vi "PositionToReceivePassSkill.vi"(5 "first call":bool, 7 "Striker/2ndStriker":enum16{"2ndStriker", "Striker"}(ring), 8 "error in (no error)":errorcluster, 9 "Robot":refnum<class "Robot.lvclass">, 10 "Game":refnum<class "Game.lvclass">, 11 "PositionToReceivePassSkill in":refnum<class "PositionToReceivePassSkill.lvclass">) -> (0 "error out":errorcluster, 2 "Robot out":refnum<class "Robot.lvclass">, 3 "PositionToReceivePassSkill out":refnum<class "PositionToReceivePassSkill.lvclass">)   [LabVIEW 2018, in "PositionToReceivePassSkill.lvclass"]
uses:
  PositionToReceivePassSkill.lvclass
  Game_class/Game.lvclass
  Robot_class/Robot.lvclass
  Game_class/Game.lvclass/Game.ctl
  Parameters_class/Parameters.lvclass/Parameters.ctl
  Team_class/Team.lvclass/Team.ctl
  Object_class/Object.lvclass/Object.ctl
  Robot_class/Robot.lvclass/Robot.ctl
  Robot_class/roles.ctl
  Utilities_class/Utilities.lvclass
  Object_class/Read x.vi
  Object_class/Read y.vi
  Robot_class/Read role.vi
  Robot_class/Read orientation.vi
  Game_class/Read OffensiveTeam.vi
  Game_class/Read FieldRef.vi
  Team_class/Read RobotRef.vi
  Game_class/Read Parameters.lvclass.vi
  Parameters_class/Read AttakingOurselves.vi
  Robot_class/Write dest_x.vi
  Robot_class/Write dest_y.vi
  Robot_class/Write dest_orientation.vi
  Ally_class/Ally.lvclass
  Field_class/Field.lvclass
  Parameters_class/Parameters.lvclass
panel:
  in  "Field defense":dbl[](array[numeric])
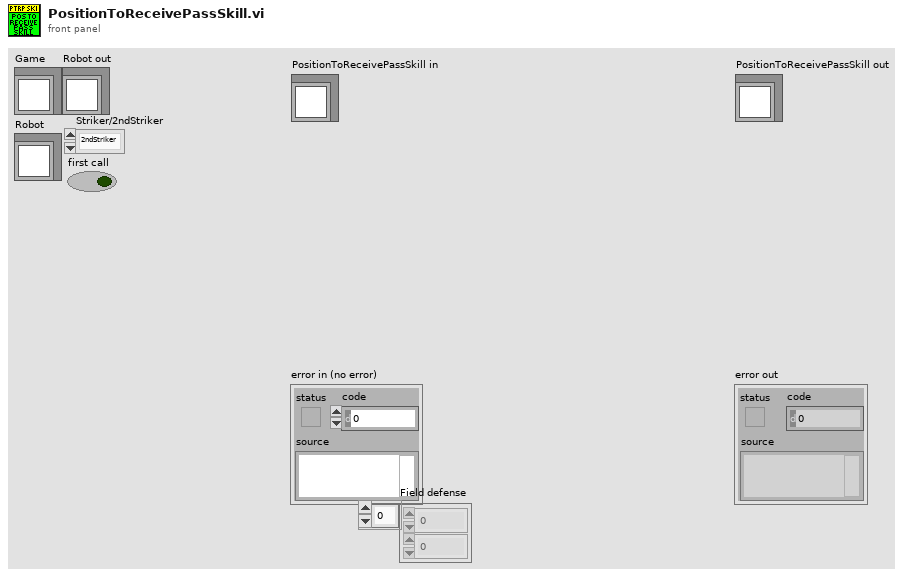
[diagram p1: front panel]
types:
  T1 = typedef "roles.ctl" = enum16{"PrepareRollToPassRoller", "PrepareRollToPassReceiver", "SimplePassRoll", "SimplePassRollReceiver", "PenaltyDefense", "PreparePassReceiver 2", "PreparePassReceiver 1", "PassObserver", "Timeout", "Goto", "ZigZag", "None", "BallOutOfField", "DefenderArea", "Duelist", "AttackerStop", "FollowAttacker", "KeeperRole", "KickPenalty", "AttackerAimGoal", "AttackerBlock", "Marker", "Halt", "Shoot", "PassKicker", "PassReceiver", "TestRole", "PenaltyAttacker"}
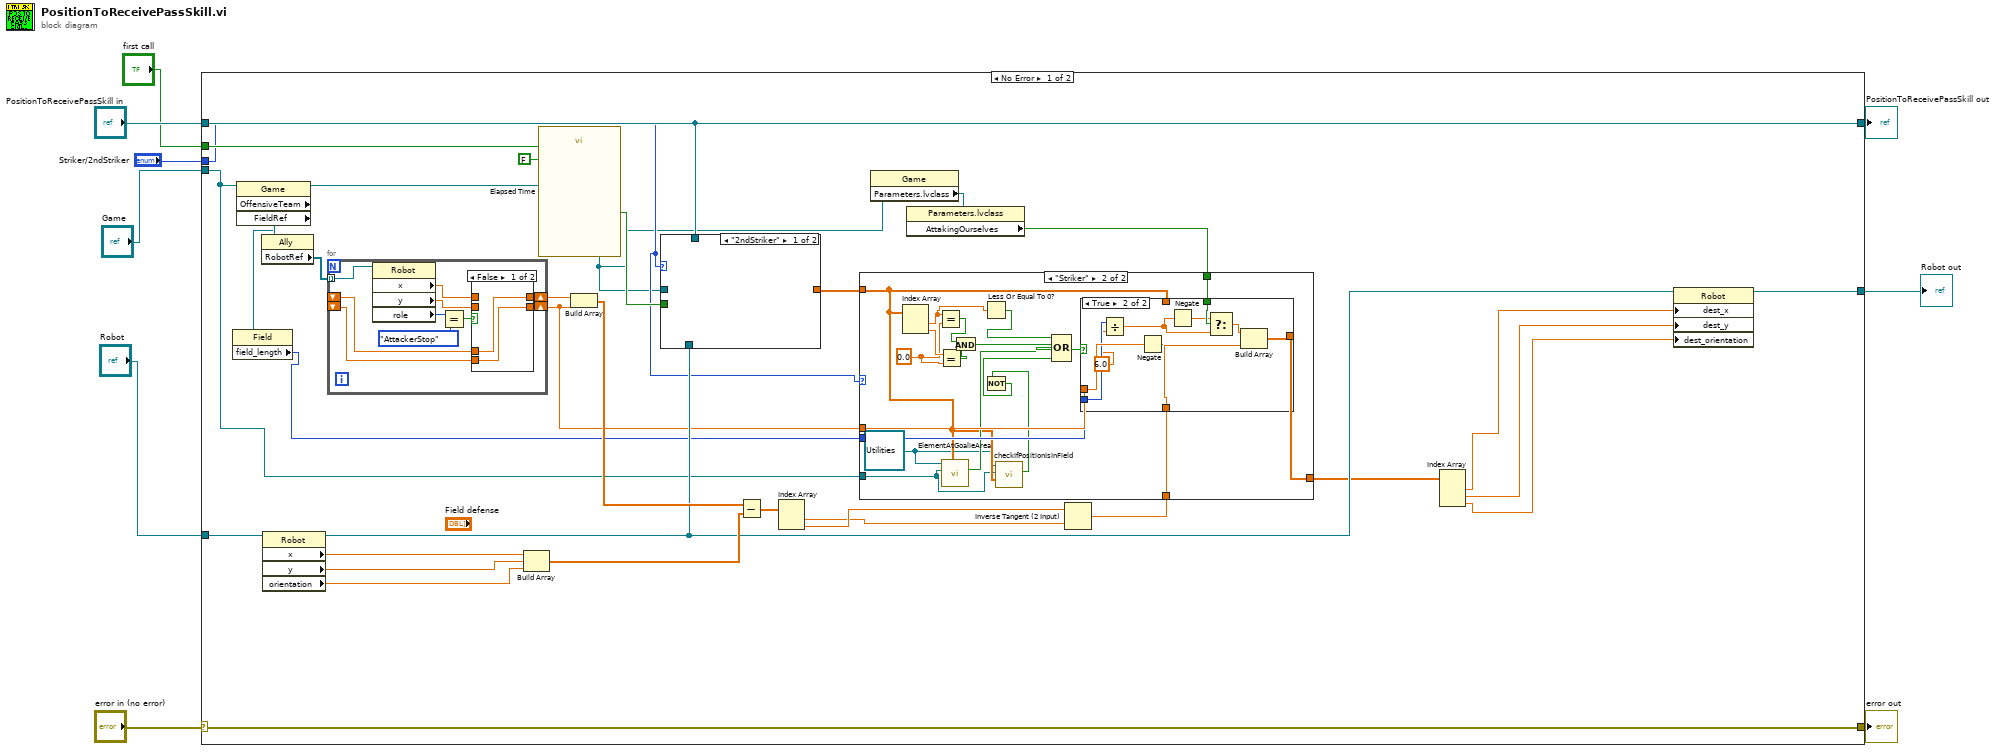
[diagram p0: block diagram]
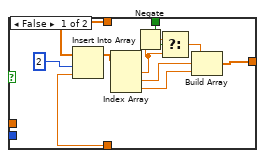
[diagram p3: hidden frame]
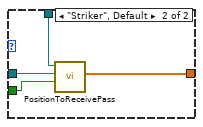
[diagram p4: hidden frame]
diagram:
  n1 = case shown="No Error" "error in (no error)" {
    selector: "error in (no error)" -> [w42 w104]
    tunnel: [w42 w104] -> w8
    tunnel: [w25 w103] -> w6
    tunnel: "PositionToReceivePassSkill in" -> [w25 w103]
    tunnel: "Game" -> [w16 _]
    tunnel: "Robot" -> [w33 w102]
    tunnel: [w29 w102] -> w3
    tunnel: "Striker/2ndStriker" -> [w15 _]
    tunnel: "first call" -> [w21 _]
    frame No Error {
      n2 = property class="Game"(reference=w16) -> (reference out=w12:refnum<class "Game.lvclass">, "OffensiveTeam"=w24:refnum<class "Ally.lvclass">, "FieldRef"=w18:refnum<class "Field.lvclass">)  [unwired: 1 in, 1 out]
      n3 = property class="Field"(reference=w18) -> ("field_length"=w17:i32)  [unwired: 1 in, 2 out]
      n4 = property class="Ally"(reference=w24) -> ("RobotRef"=w36:refnum<class "Robot.lvclass">[])  [unwired: 1 in, 2 out]
      n5 = property class="Robot"(reference=w33) -> (reference out=w23:refnum<class "Robot.lvclass">, "x"=w32:dbl, "y"=w31:dbl, "orientation"=w30:dbl)  [unwired: 1 in, 1 out]
      n6 = for {
        tunnel: w36 -> [w97] mode=indexing
        shift-right: [w91] -> w19
        shift-left: _ -> [w88]
        shift-right: [w93] -> w35
        shift-left: _ -> [w89]
        n7 = property class="Robot"(reference=w97) -> ("x"=w92:dbl, "y"=w90:dbl, "role"=w96:T1)  [unwired: 1 in, 2 out]
        n8 = Equal?(x=w96, y=roles."AttackerStop") -> (x = y?=w94:bool)
        n9 = case shown="False" w94 {
          tunnel: [w99 w101] -> w93
          tunnel: w92 -> [_ w101]
          tunnel: [w98 w100] -> w91
          tunnel: w90 -> [_ w100]
          tunnel: w89 -> [w99 _]
          tunnel: w88 -> [w98 _]
          frame False {
          }
          frame True {
          }
        }
      }
      n10 = Build Array(w32, w31, w30) -> (w37:dbl[])
      n11 = call "Elapsed Time"("Reset"=w21, "Auto Reset"=FALSE) -> ("Time has Elapsed"=w20:bool)  [unwired: 10 in, 7 out]
      n12 = Build Array(w35, w19) -> (w34:dbl[])
      n13 = case shown="\"2ndStriker\"" w15 {
        tunnel: w25 -> [_ w87]
        tunnel: w12 -> [_ w86]
        tunnel: [_ w85] -> w14
        tunnel: w23 -> [_ _]
        tunnel: w20 -> [_ w84]
        frame "2ndStriker" {
        }
        frame "Striker", Default {
          n14 = call-dynamic "PositionToReceivePass.vi"("Time Elapsed?"=w84, "Game"=w86, "PositionToReceivePassSkill in"=w87) -> ("Position"=w85:dbl[])  [unwired: 6 in, 2 out]
        }
      }
      n15 = Subtract(x=w34, y=w37) -> (x-y=w41:dbl[])
      n16 = Index Array(array=w41) -> (element #1=w39:dbl, element #2=w40:dbl)  [unwired: 2 in]
      n17 = property class="Game"(reference=w12) -> ("Parameters.lvclass"=w11:refnum<class "Parameters.lvclass">)  [unwired: 1 in, 2 out]
      n18 = property class="Parameters.lvclass"(reference=w11) -> ("AttakingOurselves"=w10:bool)  [unwired: 1 in, 2 out]
      n19 = Inverse Tangent (2 Input)(1:w39, 2:w40) -> (0:w38:dbl)
      n20 = case shown="\"Striker\"" w15 {
        tunnel: w38 -> [_ w62]
        tunnel: [w43 w61] -> w13
        tunnel: w19 -> [_ w53]
        tunnel: w17 -> [_ w52]
        tunnel: w14 -> [w43 w48]
        tunnel: w16 -> [_ w46]
        tunnel: w10 -> [_ w44]
        frame "2ndStriker", Default {
        }
        frame "Striker" {
          w47 = refnum<class "Utilities.lvclass"> refnum ("Utilities in")
          w58 = 0.0
          n21 = Index Array(array=w48) -> (element #1=w56:dbl, element #2=w59:dbl)  [unwired: 2 in]
          n22 = Equal?(x=w56, y=w58) -> (x = y?=w60:bool)
          n23 = Equal?(x=w59, y=w58) -> (x = y?=w51:bool)
          n24 = call-dynamic "ElementAtGoalieArea.vi"("Elemento pos."=w48, "Game"=w46, "Utilities in"=w47) -> ("Elemento at goalkeeper area ?"=w50:bool)  [unwired: 6 in, 2 out]
          n25 = And(x=w60, y=w51) -> (x .and. y?=w57:bool)
          n26 = Less Or Equal To 0?(x=w56) -> (x <= 0?=w54:bool)
          n27 = call "checkIfPositionIsInField.vi"("Position"=w48, "Game"=w46, "Utilities in"=w47) -> ("Position Is In Field?"=w45:bool)  [unwired: 6 in, 2 out]
          n28 = Not(x=w45) -> (.not. x?=w49:bool)
          n29 = Compound Arithmetic op=OR(w54, w57, w50, w49) -> (w55:bool)
          n30 = case shown="True" w55 {
            tunnel: w62 -> [w73 w83]
            tunnel: [w69 w82] -> w61
            tunnel: w48 -> [w71 _]
            tunnel: w53 -> [_ w80]
            tunnel: w52 -> [_ w79]
            tunnel: w44 -> [w65 w76]
            frame False {
              n31 = Insert Into Array(array=w71, index=2, new element=w73) -> (w70:dbl[])
              n32 = Index Array(array=w70) -> (element #1=w63:dbl, element #2=w68:dbl, element #3=w67:dbl)  [unwired: 3 in]
              n33 = Negate(x=w63) -> (-x=w64:dbl)
              n34 = Select(t=w64, s=w65, f=w63) -> (s? t:f=w66:dbl)
              n35 = Build Array(w66, w68, w67) -> (w69:dbl[])
            }
            frame True {
              n36 = Divide(x=w79, y=6.0) -> (x/y=w75:dbl)
              n37 = Negate(x=w80) -> (-x=w81:dbl)
              n38 = Negate(x=w75) -> (-x=w74:dbl)
              n39 = Select(t=w74, s=w76, f=w75) -> (s? t:f=w77:dbl)
              n40 = Build Array(w77, w81, w83) -> (w82:dbl[])
            }
          }
        }
      }
      n41 = Index Array(array=w13) -> (element #1=w28:dbl, element #2=w27:dbl, element #3=w26:dbl)  [unwired: 3 in]
      n42 = property class="Robot"(reference=w23, "dest_x"=w28, "dest_y"=w27, "dest_orientation"=w26) -> (reference out=w29:refnum<class "Robot.lvclass">)  [unwired: 1 in, 1 out]
    }
    frame Error {
    }
  }
  "error out" <- w8
  "PositionToReceivePassSkill out" <- w6
  "Robot out" <- w3
